vi "iniit.vi"(8 "error in (no error)":errorcluster, 11 "Controller in":refnum<class "Controller.lvclass">) -> (0 "error out":errorcluster, 3 "Controller out":refnum<class "Controller.lvclass">)   [LabVIEW 2015, in "Controller.lvclass"]
uses:
  Temperature Controller/Controller.lvclass
  Temperature Controller/Mercury Temperature Controller.lvclass
  Temperature Controller/Controller.lvclass/Controller.ctl
  <vilib>/ActorFramework/Actor/Actor.lvclass
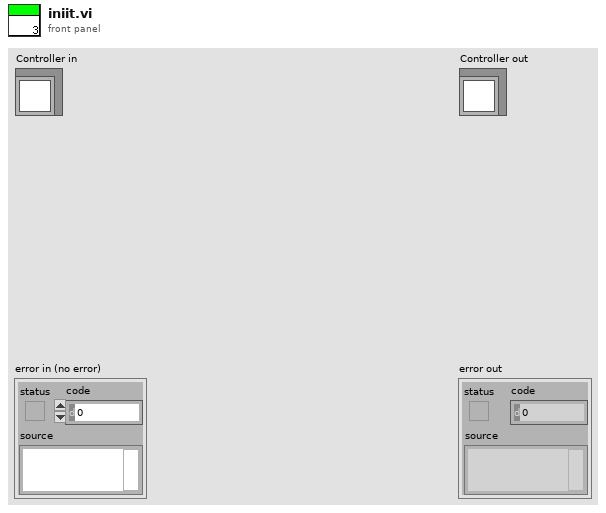
[diagram p1: front panel]
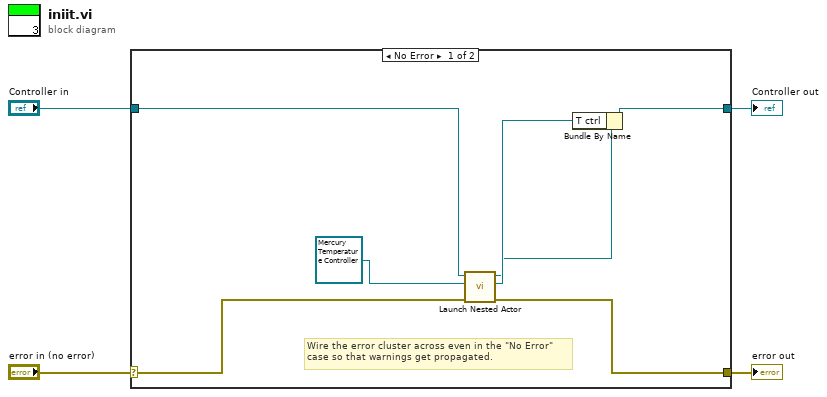
[diagram p0: block diagram]
diagram:
  n1 = case shown="No Error" "error in (no error)" {
    selector: "error in (no error)" -> [w6 w13]
    tunnel: [w5 w13] -> w3
    tunnel: [w9 w12] -> w1
    tunnel: "Controller in" -> [w10 w12]
    frame No Error {
      # "Wire the error cluster across even in the \"No Error\"\ncase so that warnings get propagated."
      n2 = call <vilib>:"Launch Nested Actor.vi"("error in (no error)"=w6, "Nested Actor"=refnum<class "Mercury Temperature Controller.lvclass"> refnum ("Mercury Temperature Controller.lvclass"), "Caller Actor in"=w10) -> ("error out"=w5:errorcluster, "Nested Actor's Enqueuer"=w8:refnum<class "Message Enqueuer.lvclass">, "Caller Actor out"=w7:refnum<class "Controller.lvclass">)  [unwired: 6 in]
      n3 = Bundle By Name(cluster=w7, "T ctrl"=w8) -> (w9:refnum<class "Controller.lvclass">)
    }
    frame Error {
    }
  }
  "error out" <- w3
  "Controller out" <- w1
